vi "CompilerCreatePulseArray.vi"(1 "step #":i32, 2 "Pulse Seq In":T3[](array[typedef])=[{"enabled"=FALSE, "string"="", "time"=0.0, "step"=0.0, "dio"=0.0, "count"=0.0, "trigger"=0.0, "AO"=0.0}], 3 "runs":i32) -> (0 "Pulse Seq Out":T1)   [LabVIEW 2019]
uses:
  SinglePulse.ctl
panel:
  in  "runs cluster":T2={"# of runs"=0, "Line trig"=TRUE, "step #"=0, "save photon times"=FALSE, "camera?"=FALSE, "# images /run"=0}
  out "AOs":u8[](array[numeric])
  out "Triggers":u8[](array[numeric])
  out "VFG times":dbl[](array[numeric])
  out "Pulses":u64[](array[numeric])
  out "Counts":u8[](array[numeric])
  out "Times":u32[](array[numeric])
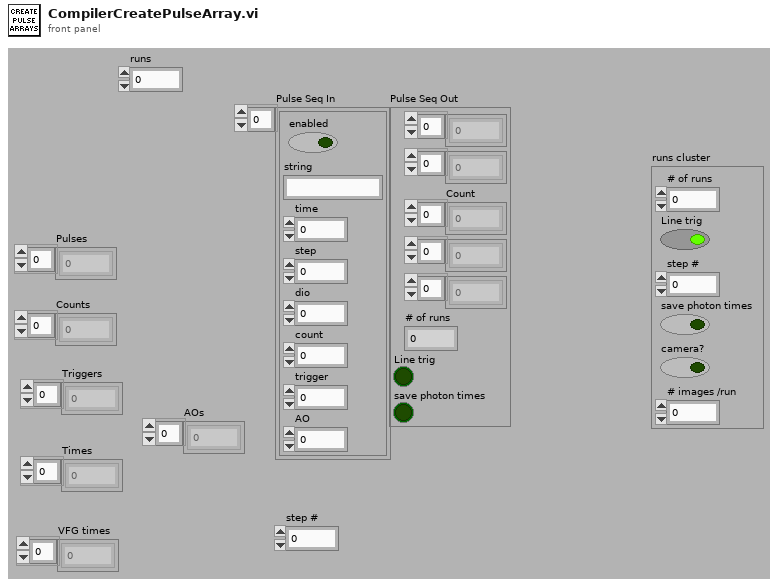
[diagram p1: front panel]
types:
  T1 = cluster{u32[], dbl[], "Count":dbl[], dbl[], dbl[], "# of runs":i32, "Line trig":bool, "save photon times":bool}
  T2 = cluster{"# of runs":i32, "Line trig":bool, "step #":i32, "save photon times":bool, "camera?":bool, "# images /run":i8}
  T3 = typedef "SinglePulse.ctl" = cluster{"enabled":bool, "string":string, "time":dbl, "step":dbl, "dio":dbl, "count":dbl, "trigger":dbl, "AO":dbl}
  T4 = cluster{u32[], dbl[], "Count":dbl[], dbl[], dbl[], "runs":i32, "Line trig":bool, "save photon times":bool}
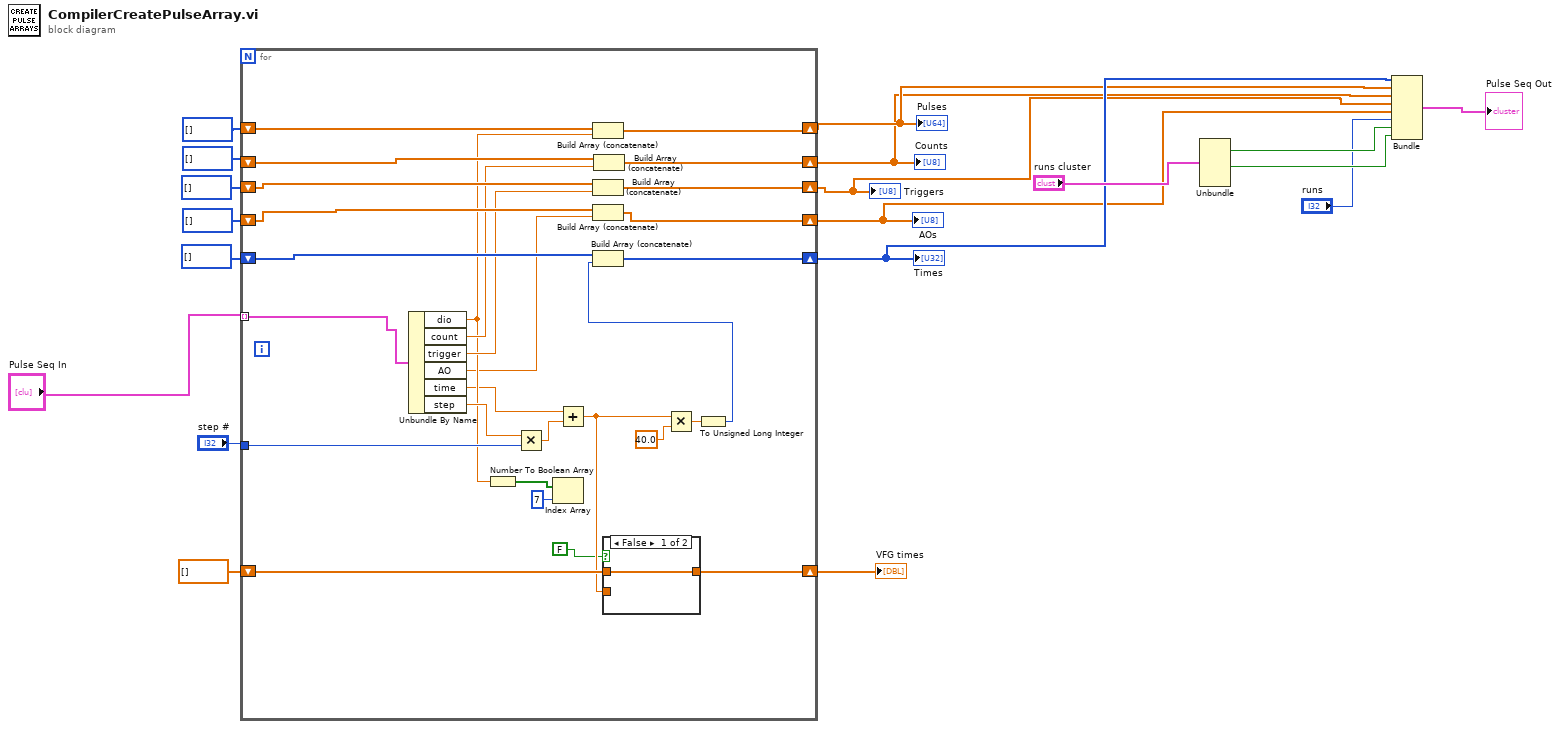
[diagram p0: block diagram]
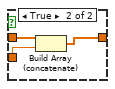
[diagram p2: hidden frame]
diagram:
  n1 = for {
    tunnel: "Pulse Seq In" -> [w21] mode=indexing
    shift-right: [w44] -> w4
    shift-left: u8[] [] -> [w47]
    shift-right: [w46] -> w7
    shift-left: u32[] [] -> [w45]
    shift-right: [w43] -> w5
    shift-left: u8[] [] ("Count") -> [w42]
    tunnel: "step #" -> [w41]
    shift-right: [w39] -> w14
    shift-left: dbl[] [] -> [w40]
    shift-right: [w37] -> w6
    shift-left: u64[] [] -> [w38]
    shift-right: [w35] -> w3
    shift-left: u8[] [] -> [w36]
    n2 = Unbundle By Name(w21) -> ("dio"=w24:dbl, "count"=w26:dbl, "trigger"=w25:dbl, "AO"=w22:dbl, "time"=w23:dbl, "step"=w27:dbl)
    n3 = Number To Boolean Array(number=w24) -> (Boolean array=w29:bool[])
    n4 = Multiply(x=w27, y=w41) -> (x*y=w34:dbl)
    n5 = Index Array(array=w29, index=7) -> ()  [unwired: 1 out]
    n6 = Add(x=w23, y=w34) -> (x+y=w28:dbl)
    n7 = Build Array (concatenate)(w38, w24) -> (w37:dbl[])
    n8 = Build Array (concatenate)(w47, w25) -> (w44:dbl[])
    n9 = Build Array (concatenate)(w36, w22) -> (w35:dbl[])
    n10 = Build Array (concatenate)(w42, w26) -> (w43:dbl[])
    n11 = case shown="False" FALSE {
      tunnel: w40 -> [w48 w50]
      tunnel: w28 -> [_ w51]
      tunnel: [w48 w49] -> w39
      frame False {
      }
      frame True {
        n12 = Build Array (concatenate)(w50, w51) -> (w49:dbl[])
      }
    }
    n13 = Multiply(x=w28, y=40.0) -> (x*y=w32:dbl)
    n14 = To Unsigned Long Integer(number=w32) -> (unsigned 32bit integer=w31:u32)
    n15 = Build Array (concatenate)(w45, w31) -> (w46:u32[])
  }
  "Times" <- w7
  "Counts" <- w5
  "Pulses" <- w6
  "VFG times" <- w14
  "Triggers" <- w4
  "AOs" <- w3
  n16 = Unbundle("runs cluster") -> ("Line trig"=w10:bool, "save photon times"=w9:bool)  [unwired: 4 out]
  n17 = Bundle(w7, w6, "Count"=w5, w4, w3, "runs"="runs", "Line trig"=w10, "save photon times"=w9) -> (→"Pulse Seq Out":T4)  [unwired: 1 in]
